vi "KepcoDCPwr Query Output Enabled.vi"(0 "VISA Session":refnum<visa-resource-name>, 5 "Model In":string, 7 "channel name (\"\")":string="\"\"", 11 "error in (no error)":errorcluster {"code" format="%.0x"}) -> (4 "VISA Session Out":refnum<visa-resource-name>, 6 "Model Out":string, 8 "channel name out (\"\")":string="\"\"" caption="channel name Out (\"\")", 12 "On":bool, 14 "Off":bool, 15 "error out":errorcluster {"code" format="%.0x"})   [LabVIEW 2013]
doc: "Inidcates if Outptu is on or off.\nWhen off, the power supply is outputing 0 volts or0 amps ."
uses:
  <vilib>/regexp/Match Regular Expression.xnode
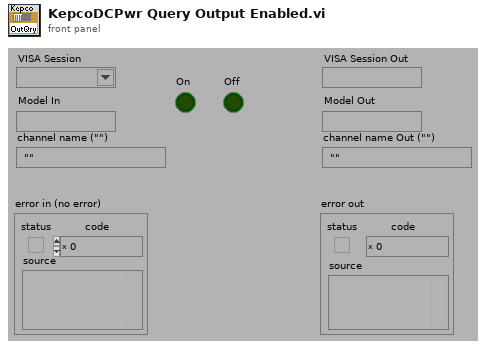
[diagram p1: front panel]
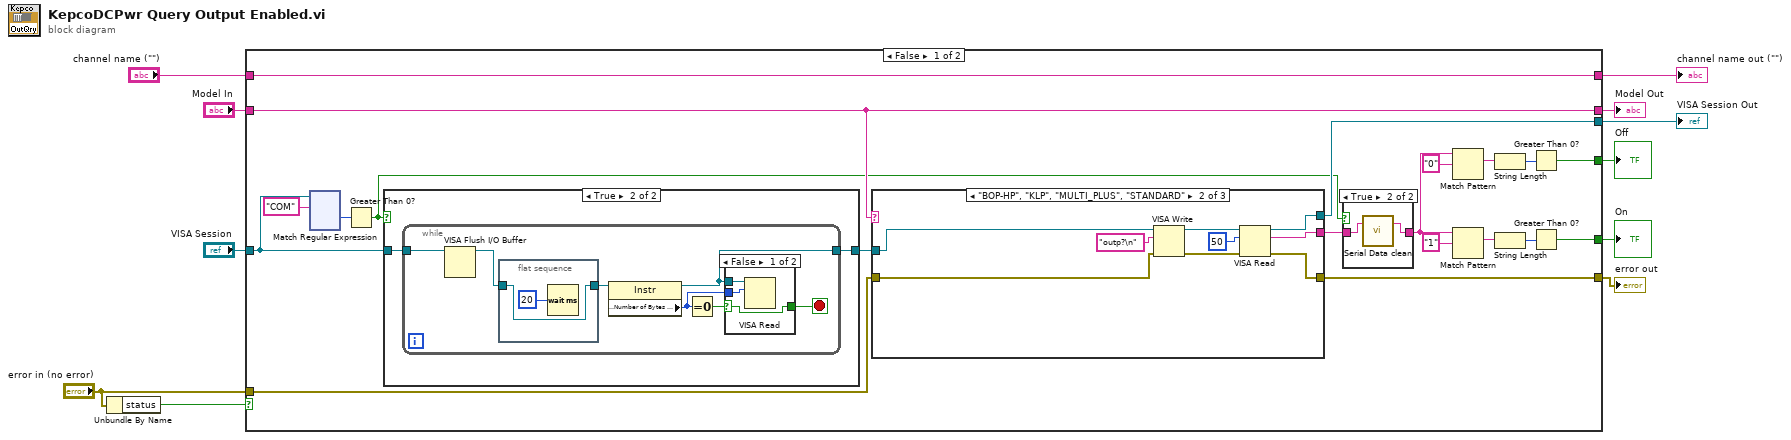
[diagram p0: block diagram]
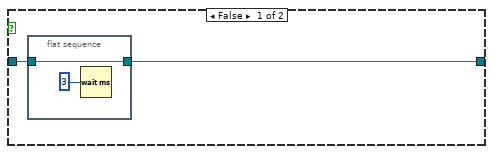
[diagram p3: hidden frame]
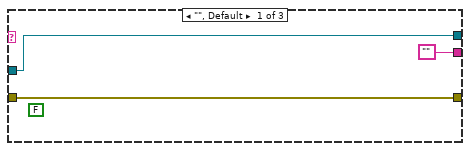
[diagram p5: hidden frame]
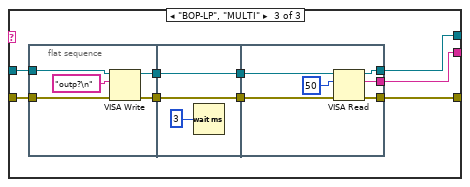
[diagram p6: hidden frame]
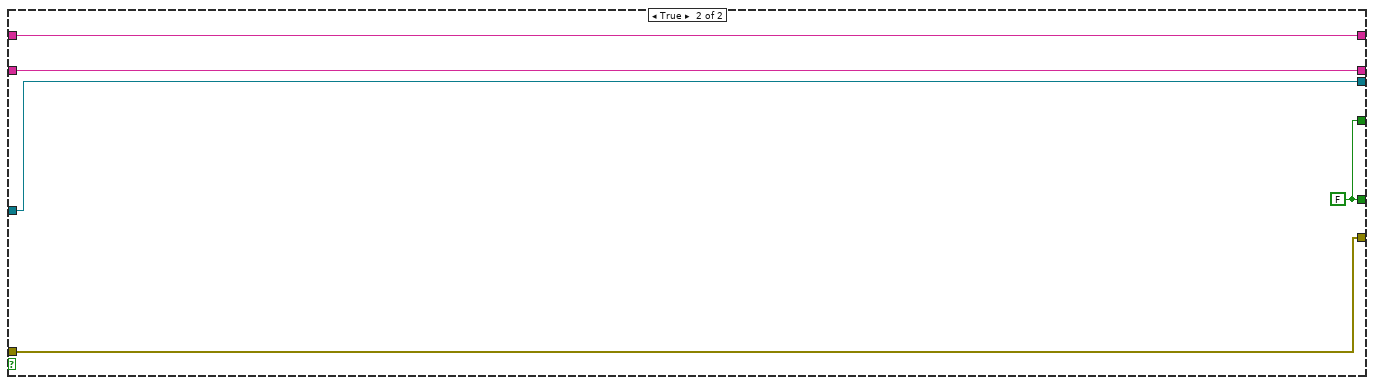
[diagram p7: hidden frame]
diagram:
  n1 = Unbundle By Name("error in (no error)") -> ("status"=w9:bool)
  n2 = case shown="False" w9 {
    tunnel: [w29 w204] -> w11
    tunnel: "error in (no error)" -> [w27 w204]
    tunnel: [w30 w200] -> w1
    tunnel: "VISA Session" -> [w16 w200]
    tunnel: "Model In" -> [w28 w203]
    tunnel: [w28 w203] -> w6
    tunnel: "channel name (\"\")" -> [w31 w202]
    tunnel: [w31 w202] -> w4
    tunnel: [w20 w201] -> w3
    tunnel: [w19 w201] -> w2
    frame False {
      n3 = xnode "Match Regular Expression"("input string"=w16, "regular expression"="COM") -> ("offset past match"=w17:i32)  [unwired: 2 in, 6 out]
      n4 = Greater Than 0?(x=w17) -> (x > 0?=w14:bool)
      n5 = case shown="True" w14 {
        tunnel: [w36 w40] -> w15
        tunnel: w16 -> [w35 w39]
        frame False {
          n6 = flat-sequence {
            tunnel: w35 -> [w38]
            tunnel: [w38] -> w36
            frame #0 {
              n7 = Wait (ms)(milliseconds to wait=u32 3 ("byte count (0)")) -> ()  [unwired: 1 out]
            }
          }
        }
        frame True {
          n8 = while {
            tunnel: w39 -> [w43]
            tunnel: [w45] -> w40
            stop <- w46 stop-if-true
            n9 = VISA Flush I/O Buffer(VISA resource name=w43) -> (VISA resource name out=w42:refnum<visa-resource-name>)  [unwired: 2 in, 1 out]
            n10 = flat-sequence {
              tunnel: w42 -> [w48]
              tunnel: [w48] -> w41
              frame #0 {
                n11 = Wait (ms)(milliseconds to wait=u32 20) -> ()  [unwired: 1 out]
              }
            }
            n12 = property class="Instr"(reference=w41) -> (reference out=w45:refnum<visa-resource-name>, "Serial Settings:Number of Bytes at Serial Port"=w44:u32)  [unwired: 1 in, 1 out]
            n13 = Equal To 0?(x=w44) -> (x = 0?=w47:bool)
            n14 = case shown="False" w47 {
              selector: w47 -> [w52 w53]
              tunnel: [w52 w53] -> w46
              tunnel: w45 -> [w51 _]
              tunnel: w44 -> [w50 _]
              frame False {
                n15 = VISA Read(VISA resource name=w51, byte count=w50) -> ()  [unwired: 1 in, 4 out]
              }
              frame True {
              }
            }
          }
        }
      }
      n16 = case shown="\"BOP-HP\", \"KLP\", \"MULTI_PLUS\", \"STANDARD\"" w28 {
        tunnel: [w167 w171 w180] -> w29
        tunnel: w15 -> [w166 w168 w177]
        tunnel: [w166 w170 w179] -> w30
        tunnel: w27 -> [w167 w174 w181]
        tunnel: ["" w169 w178] -> w13
        frame "", Default {
          (unwired) FALSE
        }
        frame "BOP-HP", "KLP", "MULTI_PLUS", "STANDARD" {
          n17 = VISA Write(VISA resource name=w168, write buffer="outp?\n", error in (no error)=w174) -> (VISA resource name out=w176:refnum<visa-resource-name>, error out=w175:errorcluster)  [unwired: 1 out]
          n18 = VISA Read(VISA resource name=w176, byte count=50, error in (no error)=w175) -> (VISA resource name out=w170:refnum<visa-resource-name>, read buffer=w169:string, error out=w171:errorcluster)  [unwired: 1 out]
        }
        frame "BOP-LP", "MULTI" {
          n19 = flat-sequence {
            tunnel: w181 -> [w190]
            tunnel: [w189] -> w185
            tunnel: [w187] -> w184
            tunnel: w177 -> [w186]
            tunnel: w185 -> [w193]
            tunnel: [w193] -> w183
            tunnel: [w192] -> w182
            tunnel: w184 -> [w192]
            tunnel: w183 -> [w198]
            tunnel: [w197] -> w180
            tunnel: w182 -> [w196]
            tunnel: [w195] -> w178
            tunnel: [w194] -> w179
            frame #0 {
              n20 = VISA Write(VISA resource name=w186, write buffer="outp?\n", error in (no error)=w190) -> (VISA resource name out=w187:refnum<visa-resource-name>, error out=w189:errorcluster)  [unwired: 1 out]
            }
            frame #1 {
              n21 = Wait (ms)(milliseconds to wait=3) -> ()  [unwired: 1 out]
            }
            frame #2 {
              n22 = VISA Read(VISA resource name=w196, byte count=50, error in (no error)=w198) -> (VISA resource name out=w194:refnum<visa-resource-name>, read buffer=w195:string, error out=w197:errorcluster)  [unwired: 1 out]
            }
          }
        }
      }
      n23 = case shown="True" w14 {
        tunnel: [w32 w33] -> w12
        tunnel: w13 -> [w32 w34]
        frame False {
        }
        frame True {
          n24 = call "Serial Data clean.vi"("string"=w34) -> ("Stripped of Xon Xoff"=w33:string)  [unwired: 2 in]
        }
      }
      n25 = Match Pattern(string=w12, regular expression="0") -> (match substring=w26:string)  [unwired: 4 out]
      n26 = Match Pattern(string=w12, regular expression="1") -> (match substring=w23:string)  [unwired: 4 out]
      n27 = String Length(string=w26) -> (length=w25:i32)
      n28 = String Length(string=w23) -> (length=w22:i32)
      n29 = Greater Than 0?(x=w25) -> (x > 0?=w20:bool)
      n30 = Greater Than 0?(x=w22) -> (x > 0?=w19:bool)
    }
    frame True {
      w201 = FALSE
    }
  }
  "error out" <- w11
  "VISA Session Out" <- w1
  "Model Out" <- w6
  "channel name out (\"\")" <- w4
  "On" <- w2
  "Off" <- w3
